vi "CustomTemplateCheck.vi"(10 "ClassTemplate":path, 11 "ClassWriterNative in":refnum<class "ClassWriterNative.lvclass">) -> (2 "ClassTemplate(Maybe Modified if not exists)":path)   [LabVIEW 2020, in "ClassWriterNative.lvclass"]
uses:
  <resource>/Framework/Providers/Open_GDS/ClassProviders/Provider_LvNativeClass/ClassWriterNative_class/ClassWriterNative.lvclass
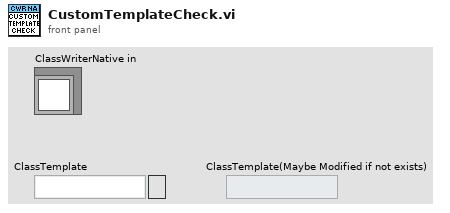
[diagram p1: front panel]
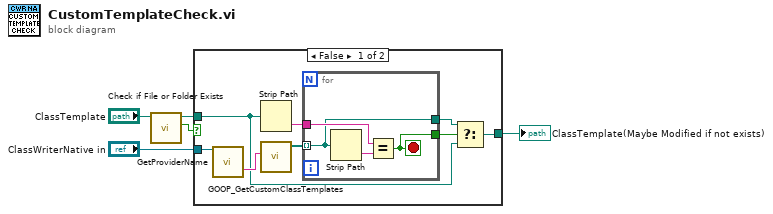
[diagram p0: block diagram]
diagram:
  n1 = call <vilib>:"Check if File or Folder Exists.vi"("path"="ClassTemplate") -> ("file or folder exists?"=w2:bool, "dup path"=w3:path)  [unwired: 8 in, 1 out]
  n2 = case shown="False" w2 {
    tunnel: "ClassWriterNative in" -> [w12 _]
    tunnel: w3 -> [w7 w18]
    tunnel: [w6 w18] -> w5
    frame False {
      n3 = call-dynamic "GetProviderName.vi"("ClassWriterNative in"=w12) -> ("ShortName(Could be used in for INI Sections)"=w13:string)  [unwired: 14 in, 4 out]
      n4 = Strip Path(path=w7) -> (name=w10:string)  [unwired: 1 out]
      n5 = call <resource>:"GOOP_GetCustomClassTemplates.vi"("ClassType"=w13) -> ("CustomTemplates"=w11:path[])  [unwired: 10 in]
      n6 = for {
        tunnel: w11 -> [w14] mode=indexing
        tunnel: w10 -> [w16]
        tunnel: [w15] -> w9
        tunnel: [w14] -> w8
        stop <- w15 stop-if-true
        n7 = Strip Path(path=w14) -> (name=w17:string)  [unwired: 1 out]
        n8 = Equal?(x=w16, y=w17) -> (x = y?=w15:bool)
      }
      n9 = Select(t=w8, s=w9, f=w7) -> (s? t:f=w6:path)
    }
    frame True {
    }
  }
  "ClassTemplate(Maybe Modified if not exists)" <- w5
